vi "DataNodeUI.vi"() -> ()   [LabVIEW 2013, in "xceDataNode.lvclass"]
doc: "Default User Interface VI."
uses:
  xceDataNode.lvclass
  <vilib>/NI/AMC/Message Queue.ctl
  <vilib>/NI/AMC/Message.ctl
  <vilib>/NI/Tools/Keyed Array/KeyedArray.ctl
  xceTreeObj/xceTreeObj.lvclass
  <vilib>/NI/AMC/Read Termination Message.vi
  <vilib>/NI/AMC/Create Single Message.vi
  <vilib>/NI/AMC/Update Message Routing Info.vi
  <vilib>/NI/AMC/Send Message.vi
  <vilib>/NI/AMC/Globals.vi
  <vilib>/NI/AMC/AMC.lvlib
  <vilib>/NI/Tools/Keyed Array/Tools_KeyedArray.lvlib
panel:
  in  "DataNode*":refnum<data-value>
  in  "AMC*":T1
  in  "Exit":bool
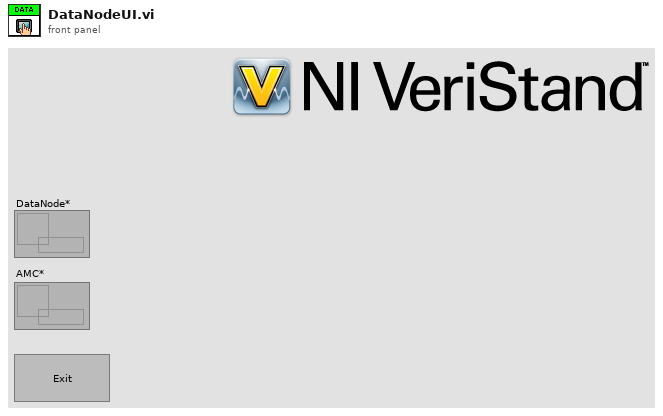
[diagram p1: front panel]
types:
  T1 = typedef "AMC.lvlib/Message Queue.ctl" = refnum<queue>
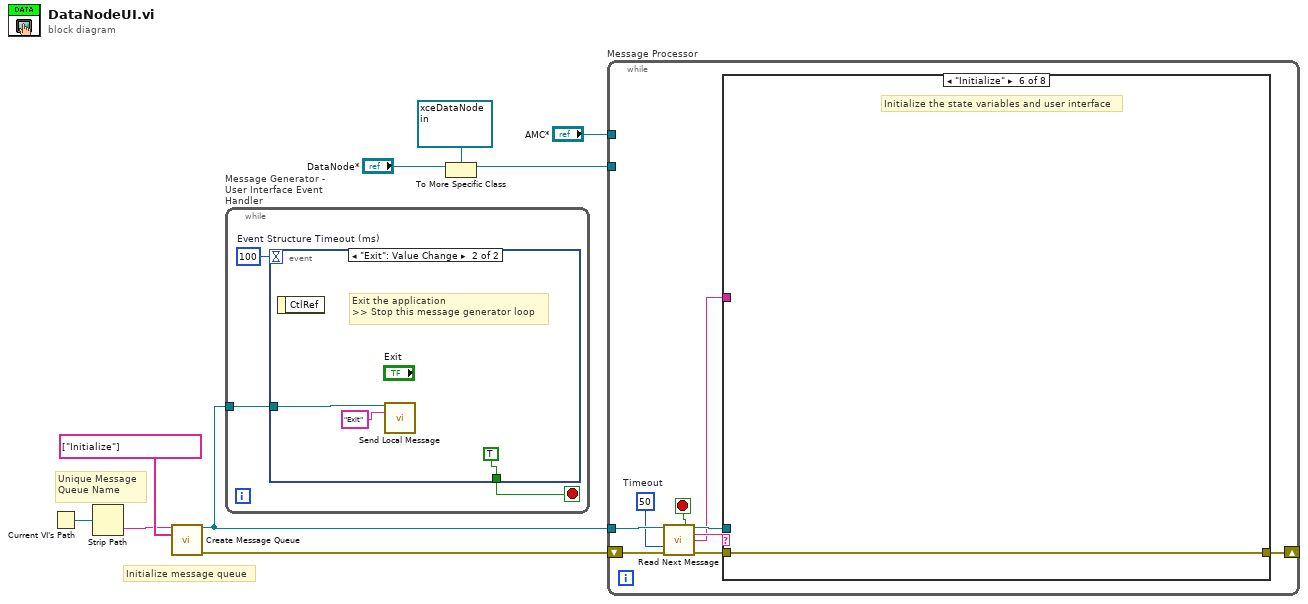
[diagram p0: block diagram]
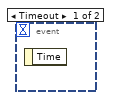
[diagram p2: hidden frame]
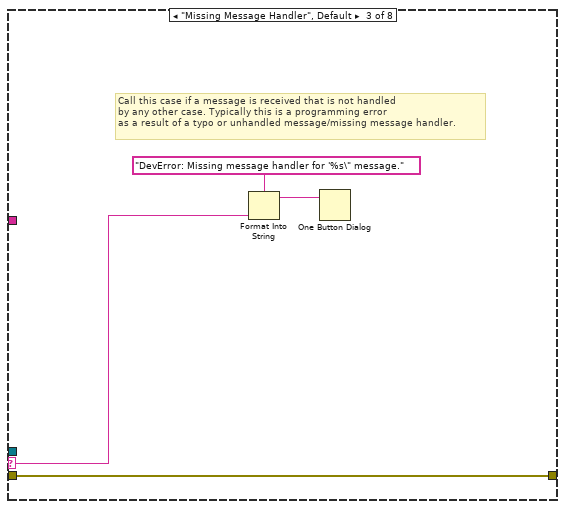
[diagram p5: hidden frame]
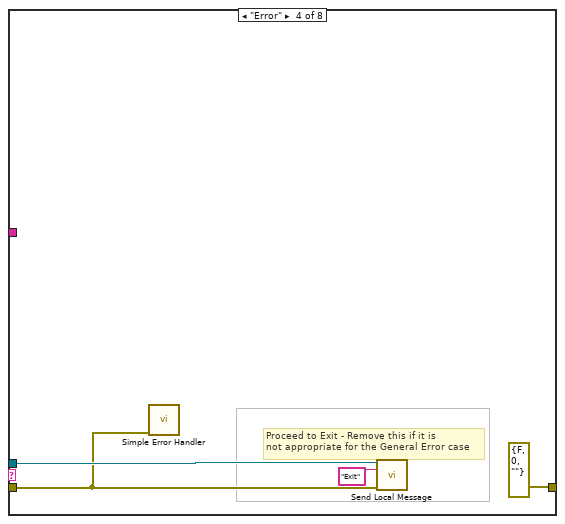
[diagram p6: hidden frame]
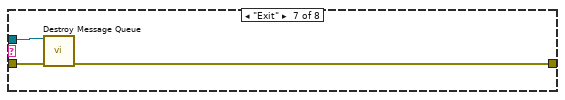
[diagram p8: hidden frame]
diagram:
  # "Initialize message queue"
  # "Unique Message\nQueue Name"
  n1 = Current VI's Path() -> (path=w5:path)
  n2 = Strip Path(path=w5) -> (name=w8:string)  [unwired: 1 out]
  n3 = call <vilib>:"Create Message Queue.vi"("message queue name"=w8, "initial message names"=string[] ["Initialize"]) -> ("message queue out"=w7:T1, "error out"=w6:errorcluster)  [unwired: 12 in]
  n4 = while "Message Generator - User Interface Event Handler" {
    tunnel: w7 -> [w10]
    stop <- w11 stop-if-true
    w12 = 100  # Event Structure Timeout (ms)
    n5 = event shown="[1] \"Exit\": Value Change" {
      selector: _ -> [_ _]
      dyn-events: _ -> [_ _]
      timeout: w12 -> [_ _]
      tunnel: [_ TRUE ("Discard?")] -> w11
      tunnel: w10 -> [_ w13]
      event Timeout {
        n6 = event-data() -> ()  [unwired: 2 out]
      }
      event "Exit": Value Change {
        # "Exit the application\n>> Stop this message generator loop"
        n7 = event-data() -> ()  [unwired: 2 out]
        n8 = call <vilib>:"Send Local Message.vi"("message queue in"=w13, "message name"="Exit") -> ()  [unwired: 11 in, 3 out]
      }
    }
  }
  n9 = To More Specific Class(target class=refnum<data-value> refnum ("DataNode*"), reference="DataNode*") -> (specific class reference=w1:refnum<data-value>)  [unwired: 1 in, 1 out]
  n10 = while "Message Processor" {
    shift-left: w6 -> [w20]
    shift-right: [w24] -> _
    tunnel: w7 -> [w21]
    tunnel: "AMC*" -> [_]
    tunnel: w1 -> [_]
    stop <- w23 stop-if-true
    w18 = 50  # Timeout
    n11 = call <vilib>:"Read Next Message.vi"("message queue in"=w21, "timeout (1 ms)"=w18, "error in"=w20) -> ("exit process?"=w23:bool, "message queue out"=w22:T1, "message name"=w17:string, "message value"=w16:string, "error out"=w19:errorcluster)  [unwired: 5 in, 3 out]
    n12 = case shown="\"Initialize\"" w17 {
      selector: w17 -> [_ _ w29 _ _ _ _ _]
      tunnel: w22 -> [_ _ _ w33 _ _ w38 _]
      tunnel: w19 -> [w25 w26 w30 w31 w35 w36 w39 w40]
      tunnel: [w25 w26 w30 errorcluster {"status"=FALSE, "code"=0, "source"=""} ("error out") w35 w36 w37 w40] -> w24
      tunnel: w16 -> [_ _ _ _ _ _ _ _]
      frame "---------- Framework Operations ----------" {
        # "Dummy case to add a seperator in the Case Structure menu"
      }
      frame "", "Idle" {
      }
      frame "Missing Message Handler", Default {
        # "Call this case if a message is received that is not handled \nby any other case. Typically this is a programming error\nas a result of a typo or unhandled message/missing message handler."
        n13 = Format Into String(format string="DevError: Missing message handler for '%s\" message." ("message"), w29) -> (resulting string=w27:string)  [unwired: 2 in, 1 out]
        n14 = One Button Dialog(message=w27) -> ()  [unwired: 2 out]
      }
      frame "Error" {
        # "Proceed to Exit - Remove this if it is\nnot appropriate for the General Error case"
        n15 = call <vilib>:"Simple Error Handler.vi"("error in (no error)"=w31) -> ()  [unwired: 1 in, 8 out]
        n16 = call <vilib>:"Send Local Message.vi"("message queue in"=w33, "message name"="Exit", "error in"=w31) -> ()  [unwired: 10 in, 3 out]
      }
      frame "---------- Generic Operations ----------" {
        # "Dummy case to add a seperator in the Case Structure menu"
      }
      frame "Initialize" {
        # "Initialize the state variables and user interface"
      }
      frame "Exit" {
        n17 = call <vilib>:"Destroy Message Queue.vi"("message queue in"=w38, "error in"=w39) -> ("error out"=w37:errorcluster)  [unwired: 11 in, 2 out]
      }
      frame "---------- Application Operations ----------" {
        # "Dummy case to add a seperator in the Case Structure menu"
      }
    }
  }
